vi "visa closed connection.vi"(8 "error in (no error)":errorcluster, 11 "simulado in":refnum<class "simulado.lvclass">) -> (0 "error out":errorcluster, 3 "simulado out":refnum<class "simulado.lvclass">)   [LabVIEW 2019, in "simulado.lvclass"]
uses:
  simulado.lvclass
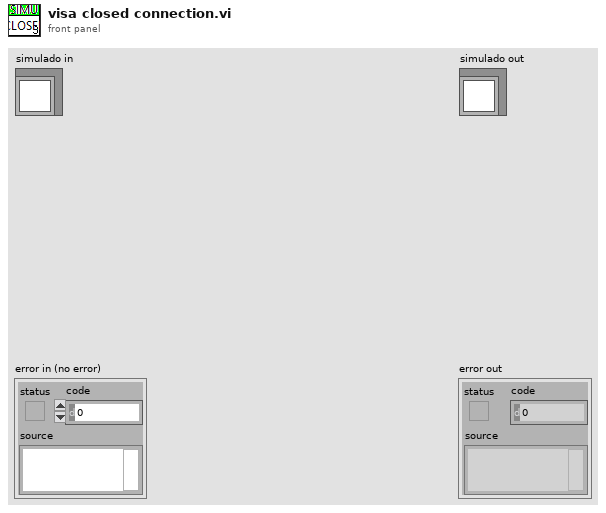
[diagram p1: front panel]
types:
  T1 = enum16{"get parameter", "Set parameters", "reset parameter", ""}
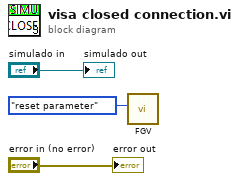
[diagram p0: block diagram]
diagram:
  n1 = call "FGV.vi"("functions"=T1."reset parameter") -> ()  [unwired: 9 in, 2 out]
  "error out" <- "error in (no error)"
  "simulado out" <- "simulado in"
